vi "逆解.vi"(6 "机械臂末端坐标":dbl[](array[numeric])=[-2177.0, 0.0, 558.0], 7 "机械臂末端姿态":dbl[][](array[numeric])=[[0.0, 0.0, -1.0], [0.0, 1.0, 0.0], [1.0, 0.0, 0.0]]) -> (0 "逆解4":dbl[](array[numeric]) format="%#.6f", 1 "逆解3":dbl[](array[numeric]) format="%#.6f", 2 "逆解2":dbl[](array[numeric]) format="%#.6f", 3 "逆解1":dbl[](array[numeric]) format="%#.6f")   [LabVIEW 2014]
uses:
  <vilib>/Utility/file.llb/Read From Spreadsheet File (DBL).vi
panel:
  out "t21":dbl
  out "z4":dbl
  out "y4":dbl
  out "x4":dbl
  out "t62":dbl
  out "t61":dbl
  out "t5":dbl
  out "t4":dbl
  out "t3":dbl
  out "t2":dbl
  out "t1":dbl
  out "角度常量":dbl
  out "弧度常量":dbl
  out "theta64":dbl
  out "theta63":dbl
  out "theta62":dbl
  out "theta61":dbl
  out "theta54":dbl
  out "theta53":dbl
  out "theta52":dbl
  out "theta51":dbl
  out "theta44":dbl
  out "theta43":dbl
  out "theta42":dbl
  out "theta41":dbl
  out "theta32":dbl
  out "theta31":dbl
  out "theta24":dbl
  out "theta23":dbl
  out "theta22":dbl
  out "theta21":dbl
  out "theta1":dbl
  out "L6":dbl
  out "L4":dbl
  out "L1":dbl
  out "L3":dbl
  out "px":dbl
  out "py":dbl
  out "pz":dbl
  out "nx":dbl
  out "ny":dbl
  out "nz":dbl
  out "az":dbl
  out "ay":dbl
  out "ax":dbl
  in  "机械臂长":dbl[](array[numeric])=[558.0, 764.0, 993.0, 420.0]
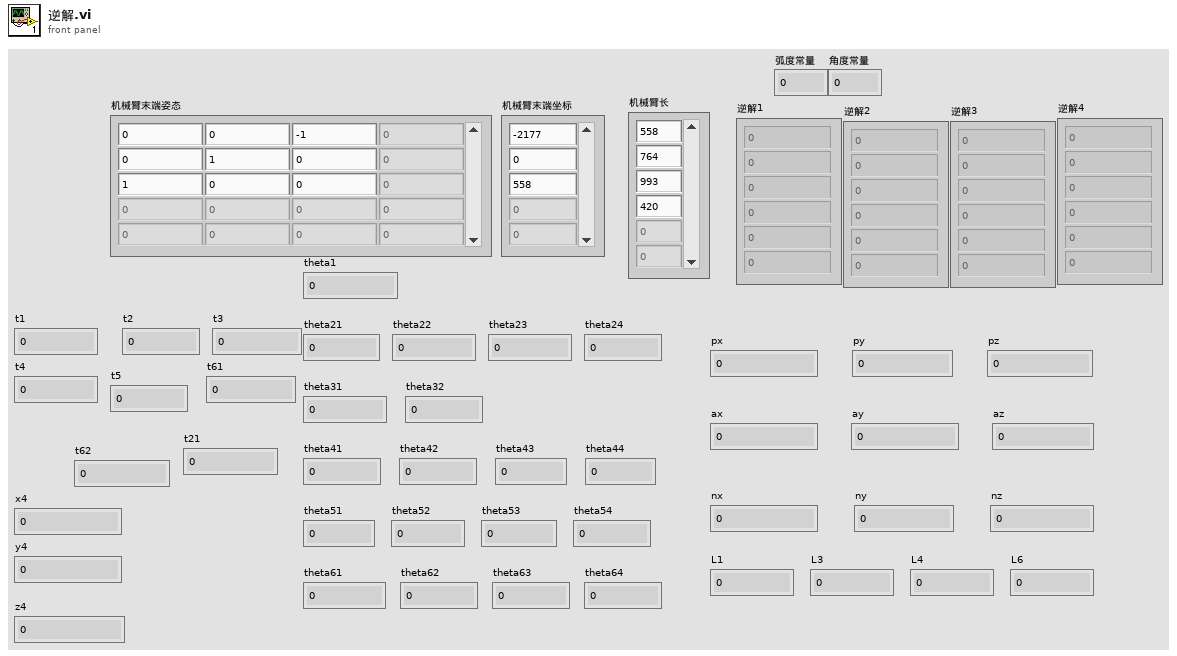
[diagram p1: front panel]
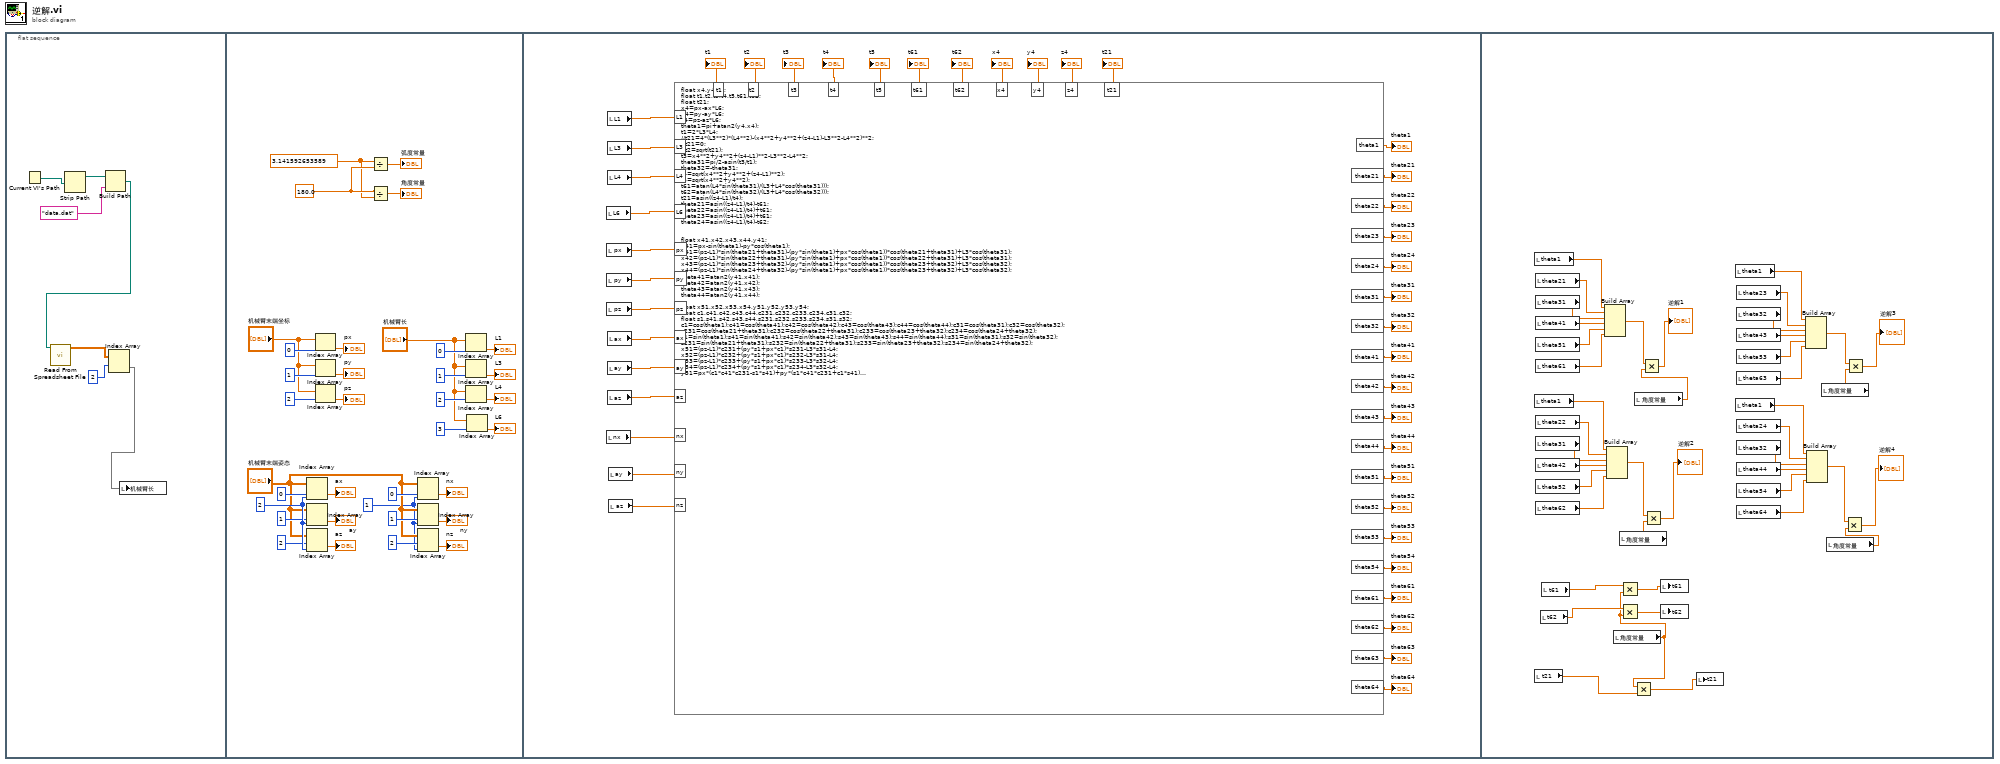
[diagram p0: block diagram]
diagram:
  n1 = flat-sequence {
    frame #0 {
      n2 = Current VI's Path() -> (path=w5:path)
      n3 = Strip Path(path=w5) -> (stripped path=w4:path)  [unwired: 1 out]
      n4 = Build Path(base path=w4, name or relative path="data.dat") -> (appended path=w2:path)
      n5 = call-poly <vilib>:"Read From Spreadsheet File.vi"("file path (dialog if empty)"=w2) -> ("all rows"=w7:dbl[][])  [unwired: 6 in, 4 out]
      n6 = Index Array(array=w7, index (row)=2) -> (element=w1:dbl[])  [unwired: 1 in]
      n7 = local write "机械臂长"(w1) -> ()
    }
    frame #1 {
      w11 = 180.0
      w10 = 3.141592653589
      w28 = 1
      w42 = 2
      n8 = Index Array(array="机械臂末端姿态", index (row)=0, index (col)=w42) -> (element=→"ax":dbl)
      n9 = Index Array(array="机械臂末端姿态", index (row)=1, index (col)=w42) -> (element=→"ay":dbl)
      n10 = Index Array(array="机械臂末端姿态", index (row)=2, index (col)=w42) -> (element=→"az":dbl)
      n11 = Index Array(array="机械臂末端坐标", index=0) -> (element=→"px":dbl)
      n12 = Index Array(array="机械臂末端坐标", index=1) -> (element=→"py":dbl)
      n13 = Index Array(array="机械臂末端坐标", index=2) -> (element=→"pz":dbl)
      n14 = Divide(x=w10, y=w11) -> (x/y=→"弧度常量":dbl)
      n15 = Divide(x=w11, y=w10) -> (x/y=→"角度常量":dbl)
      n16 = Index Array(array="机械臂末端姿态", index (row)=0, index (col)=w28) -> (element=→"nx":dbl)
      n17 = Index Array(array="机械臂末端姿态", index (row)=1, index (col)=w28) -> (element=→"ny":dbl)
      n18 = Index Array(array="机械臂末端姿态", index (row)=2, index (col)=w28) -> (element=→"nz":dbl)
      n19 = Index Array(array="机械臂长", index=0) -> (element=→"L1":dbl)
      n20 = Index Array(array="机械臂长", index=1) -> (element=→"L3":dbl)
      n21 = Index Array(array="机械臂长", index=2) -> (element=→"L4":dbl)
      n22 = Index Array(array="机械臂长", index=3) -> (element=→"L6":dbl)
    }
    frame #2 {
      n23 = local read "L6"() -> (w63:dbl)
      n24 = local read "nx"() -> (w64:dbl)
      n25 = local read "px"() -> (w62:dbl)
      n26 = local read "py"() -> (w61:dbl)
      n27 = local read "pz"() -> (w57:dbl)
      n28 = local read "L1"() -> (w54:dbl)
      n29 = local read "L3"() -> (w55:dbl)
      n30 = local read "L4"() -> (w56:dbl)
      n31 = local read "ax"() -> (w58:dbl)
      n32 = local read "ay"() -> (w59:dbl)
      n33 = local read "az"() -> (w60:dbl)
      n34 = local read "ay"() -> (w65:dbl)
      n35 = local read "az"() -> (w66:dbl)
      n36 = formula code="float x4,y4,z4;\nfloat t1,t2,t3,t4,t5,t61,t62;\nfloat t21;\nx4=px-ax*L6;\ny4=py-ay*L6;\nz4=pz-az*L6;\ntheta1=pi+atan2(y4,x4);\nt1=2*L3*L4;\n//t21=4*(L3**2)*(L4**2)-(x4**2+y4**2+(z4-L1)-L3**2-L4**2)**2;\n//t21=0;\n//t2=sqrt(t21);\nt3=x4**2+y4**2+(z4-L1)**2-L3**2-L4**2;\ntheta31=pi/2-asin(t3/t1);\ntheta32=-theta31;\nt4=sqrt(x4**2+y4**2+(z4-L1)**2);\nt5=sqrt(x4**2+y4**2);\nt61=atan(L4*sin(theta31)/(L3+L4*cos(theta31)));\nt62=atan(L4*sin(theta32)/(L3+L4*cos(theta32)));\nt21=asin((z4-L1)/t4);\ntheta21=asin((z4-L1)/t4)-t61;\ntheta22=asin((z4-L1)/t4)+t61;\ntheta23=asin((z4-L1)/t4)+t61;\ntheta24=asin((z4-L1)/t4)-t62;\n\n\nfloat x41,x42,x43,x44,y41;\ny41=px-sin(theta1)-py*cos(theta1);\nx41=(pz-L1)*sin(theta21+theta31)-(py*sin(theta1)+px*cos(theta1))*cos(theta21+theta31)+L3*cos(theta31);\nx42=(pz-L1)*sin(theta22+theta31)-(py*sin(theta1)+px*cos(theta1))*cos(theta22+theta31)+L3*cos(theta31);\nx43=(pz-L1)*sin(theta23+theta32)-(py*sin(theta1)+px*cos(theta1))*cos(theta23+theta32)+L3*cos(theta32);\nx44=(pz-L1)*sin(theta24+theta32)-(py*sin(theta1)+px*cos(theta1))*cos(theta23+theta32)+L3*cos(theta32);\ntheta41=atan2(y41,x41);\ntheta42=atan2(y41,x42);\ntheta43=atan2(y41,x43);\ntheta44=atan2(y41,x44);\n\nfloat x51,x52,x53,x54,y51,y52,y53,y54;\nfloat c1,c41,c42,c43,c44,c231,c232,c233,c234,c31,c32;\nfloat s1,s41,s42,s43,s44,s231,s232,s233,s234,s31,s32;\nc1=cos(theta1);c41=cos(theta41);c42=cos(theta42);c43=cos(theta43);c44=cos(theta44);c31=cos(theta31);c32=cos(theta32);\nc231=cos(theta21+theta31);c232=cos(theta22+theta31);c233=cos(theta23+theta32);c234=cos(theta24+theta32);\ns1=sin(theta1);s41=sin(theta41);s42=sin(theta42);s43=sin(theta43);s44=sin(theta44);s31=sin(theta31);s32=sin(theta32);\ns231=sin(theta21+theta31);s232=sin(theta22+theta31);s233=sin(theta23+theta32);s234=sin(theta24+theta32);\nx51=(pz-L1)*c231+(py*s1+px*c1)*s231-L3*s31-L4;\nx52=(pz-L1)*c232+(py*s1+px*c1)*s232-L3*s31-L4;\nx53=(pz-L1)*c233+(py*s1+px*c1)*s233-L3*s32-L4;\nx54=(pz-L1)*c234+(py*s1+px*c1)*s234-L3*s32-L4;\ny51=px*(c1*c41*c231-s1*s41)+py*(s1*c41*c231+c1*s41)+(L1-pz)*c41*s231-L3*c41*c31;\ny52=px*(c1*c42*c232-s1*s42)+py*(s1*c42*c232+c1*s42)+(L1-pz)*c42*s232-L3*c42*c31;\ny53=px*(c1*c43*c233-s1*s43)+py*(s1*c43*c233+c1*s43)+(L1-pz)*c43*s233-L3*c43*c32;\ny54=px*(c1*c44*c234-s1*s44)+py*(s1*c44*c234+c1*s44)+(L1-pz)*c44*s234-L3*c44*c32;\ntheta51=atan2(y51,x51);\ntheta52=atan2(y52,x52);\ntheta53=atan2(y53,x53);\ntheta54=atan2(y54,x54);\n\nfloat s51,s52,s53,s54;\nfloat y61,y62,y63,y64,x61,x62,x63,x64;\ns51=sin(theta51);s52=sin(theta52);s53=sin(theta53);s54=sin(theta54);\nx61=s51-nz*c231-(nx*c1+ny*s1)*s231;\nx62=s52-nz*c232-(nx*c1+ny*s1)*s232;\nx63=s53-nz*c233-(nx*c1+ny*s1)*s233;\nx64=s54-nz*c234-(nx*c1+ny*s1)*s234;\ny61=s51+nz*c231+(nx*c1+ny*s1)*s231;\ny62=s52+nz*c232+(nx*c1+ny*s1)*s232;\ny63=s53+nz*c233+(nx*c1+ny*s1)*s233;\ny64=s54+nz*c234+(nx*c1+ny*s1)*s234;\ntheta61=atan2(y61,x61);\ntheta62=atan2(y62,x62);\ntheta63=atan2(y63,x63);\ntheta64=atan2(y64,x64);"("L1"=w54, "L3"=w55, "L4"=w56, "px"=w62, "py"=w61, "pz"=w57, "ax"=w58, "ay"=w59, "az"=w60, "L6"=w63, "nx"=w64, "ny"=w65, "nz"=w66) -> ("theta1"=→"theta1":dbl, "theta21"=→"theta21":dbl, "theta22"=→"theta22":dbl, "theta23"=→"theta23":dbl, "theta24"=→"theta24":dbl, "theta31"=→"theta31":dbl, "theta32"=→"theta32":dbl, "theta41"=→"theta41":dbl, "theta42"=→"theta42":dbl, "theta43"=→"theta43":dbl, "theta44"=→"theta44":dbl, "theta51"=→"theta51":dbl, "theta52"=→"theta52":dbl, "theta53"=→"theta53":dbl, "theta54"=→"theta54":dbl, "theta61"=→"theta61":dbl, "theta62"=→"theta62":dbl, "theta63"=→"theta63":dbl, "theta64"=→"theta64":dbl, "t1"=→"t1":dbl, "t2"=→"t2":dbl, "t3"=→"t3":dbl, "t4"=→"t4":dbl, "t5"=→"t5":dbl, "t61"=→"t61":dbl, "t62"=→"t62":dbl, "x4"=→"x4":dbl, "y4"=→"y4":dbl, "z4"=→"z4":dbl, "t21"=→"t21":dbl)
    }
    frame #3 {
      n37 = local read "theta1"() -> (w105:dbl)
      n38 = local read "theta1"() -> (w116:dbl)
      n39 = local read "t21"() -> (w87:dbl)
      n40 = local read "theta21"() -> (w106:dbl)
      n41 = local read "theta31"() -> (w107:dbl)
      n42 = local read "theta41"() -> (w108:dbl)
      n43 = local read "theta51"() -> (w109:dbl)
      n44 = local read "theta61"() -> (w110:dbl)
      n45 = local read "theta22"() -> (w115:dbl)
      n46 = local read "theta31"() -> (w114:dbl)
      n47 = local read "theta42"() -> (w113:dbl)
      n48 = local read "theta52"() -> (w112:dbl)
      n49 = local read "theta62"() -> (w111:dbl)
      n50 = local read "t62"() -> (w91:dbl)
      n51 = local read "t61"() -> (w92:dbl)
      n52 = Build Array(w105, w106, w107, w108, w109, w110) -> (w103:dbl[])
      n53 = Build Array(w116, w115, w114, w113, w112, w111) -> (w97:dbl[])
      n54 = local read "角度常量"() -> (w88:dbl)
      n55 = local read "角度常量"() -> (w98:dbl)
      n56 = Multiply(x=w92, y=w88) -> (x*y=w90:dbl)
      n57 = Multiply(x=w91, y=w88) -> (x*y=w89:dbl)
      n58 = Multiply(x=w88, y=w87) -> (x*y=w86:dbl)
      n59 = local read "角度常量"() -> (w104:dbl)
      n60 = Multiply(x=w103, y=w104) -> (x*y=→"逆解1":dbl[])
      n61 = Multiply(x=w97, y=w98) -> (x*y=→"逆解2":dbl[])
      n62 = local write "t61"(w90) -> ()
      n63 = local write "t62"(w89) -> ()
      n64 = local write "t21"(w86) -> ()
      n65 = local read "theta1"() -> (w117:dbl)
      n66 = local read "theta1"() -> (w128:dbl)
      n67 = local read "theta23"() -> (w118:dbl)
      n68 = local read "theta32"() -> (w119:dbl)
      n69 = local read "theta43"() -> (w120:dbl)
      n70 = local read "theta53"() -> (w121:dbl)
      n71 = local read "theta63"() -> (w122:dbl)
      n72 = local read "theta24"() -> (w127:dbl)
      n73 = local read "theta32"() -> (w126:dbl)
      n74 = local read "theta44"() -> (w125:dbl)
      n75 = local read "theta54"() -> (w124:dbl)
      n76 = local read "theta64"() -> (w123:dbl)
      n77 = Build Array(w117, w118, w119, w120, w121, w122) -> (w100:dbl[])
      n78 = Build Array(w128, w127, w126, w125, w124, w123) -> (w94:dbl[])
      n79 = local read "角度常量"() -> (w101:dbl)
      n80 = local read "角度常量"() -> (w95:dbl)
      n81 = Multiply(x=w94, y=w95) -> (x*y=→"逆解4":dbl[])
      n82 = Multiply(x=w100, y=w101) -> (x*y=→"逆解3":dbl[])
    }
  }
